vi "Serialize File Attributes.vi"(1 "file attributes":T1 {"permissions" format="%04o"}) -> (0 "Array":u8[](array[numeric]) format="%02x")   [LabVIEW 2020, in "NI_SFTP.lvlib"]
uses:
  <vilib>/net/SFTP/NI_SFTP.lvlib
  <vilib>/net/SFTP/API/Support/File Attributes.ctl
  <vilib>/net/SFTP/Low Level Connection/Serialize U32.vi
  <vilib>/net/SFTP/Low Level Connection/Serialize Byte Array.vi
  <vilib>/net/SFTP/Low Level Connection/Serialize U64.vi
  <vilib>/net/SFTP/Low Level Connection/Low Level Connection.lvclass
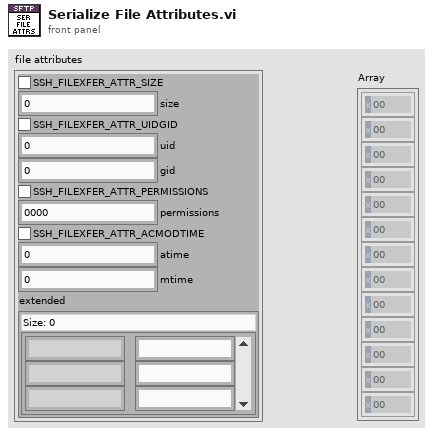
[diagram p1: front panel]
types:
  T1 = typedef "NI_SFTP.lvlib/File Attributes.ctl" = cluster{"SSH_FILEXFER_ATTR_SIZE":bool, "size":u64, "SSH_FILEXFER_ATTR_UIDGID":bool, "uid":u32, "gid":u32, "SSH_FILEXFER_ATTR_PERMISSIONS":bool, "permissions":u32, "SSH_FILEXFER_ATTR_ACMODTIME":bool, "atime":u32, "mtime":u32, "extended":map{string, string}}
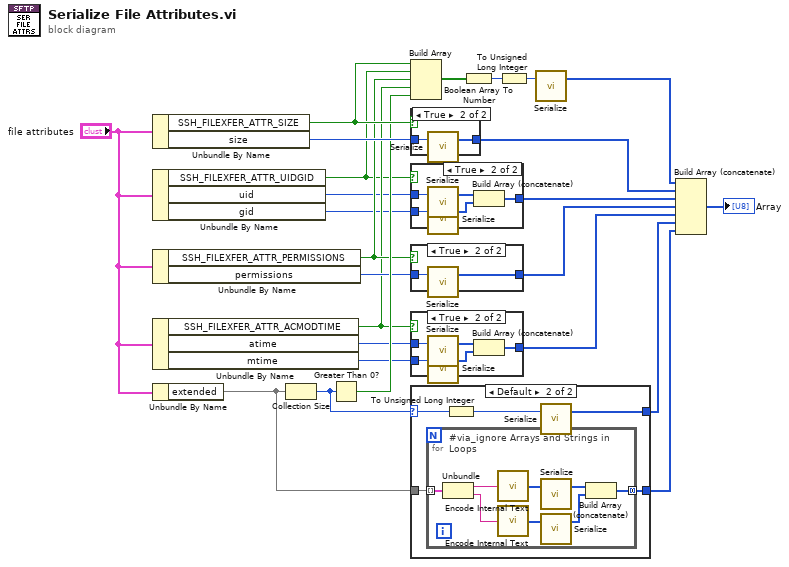
[diagram p0: block diagram]
diagram:
  n1 = Unbundle By Name("file attributes") -> ("SSH_FILEXFER_ATTR_SIZE"=w22:bool, "size"=w21:u64)
  n2 = Unbundle By Name("file attributes") -> ("SSH_FILEXFER_ATTR_UIDGID"=w6:bool, "uid"=w5:u32, "gid"=w4:u32)
  n3 = Unbundle By Name("file attributes") -> ("SSH_FILEXFER_ATTR_PERMISSIONS"=w11:bool, "permissions"=w10:u32)
  n4 = Unbundle By Name("file attributes") -> ("SSH_FILEXFER_ATTR_ACMODTIME"=w9:bool, "atime"=w8:u32, "mtime"=w7:u32)
  n5 = Unbundle By Name("file attributes") -> ("extended"=w12:map{string, string})
  n6 = Collection Size(1:w12) -> (0:w19:i32)
  n7 = Greater Than 0?(x=w19) -> (x > 0?=w20:bool)
  n8 = Build Array(w22, w6, w11, w9, w20) -> (w25:bool[])
  n9 = case shown="True" w22 {
    tunnel: w21 -> [_ w27]
    tunnel: [_ w26] -> w17
    frame False {
    }
    frame True {
      n10 = call-poly <vilib>:"Serialize.vi"("data"=w27) -> ("bytes"=w26:u8[])  [unwired: 2 in]
    }
  }
  n11 = case shown="True" w6 {
    tunnel: w5 -> [_ w32]
    tunnel: [_ w30] -> w16
    tunnel: w4 -> [_ w29]
    frame False {
    }
    frame True {
      n12 = call-poly <vilib>:"Serialize.vi"("data"=w32) -> ("bytes"=w31:u8[])  [unwired: 2 in]
      n13 = call-poly <vilib>:"Serialize.vi"("data"=w29) -> ("bytes"=w28:u8[])  [unwired: 2 in]
      n14 = Build Array (concatenate)(w31, w28) -> (w30:u8[])
    }
  }
  n15 = case shown="True" w11 {
    tunnel: w10 -> [_ w34]
    tunnel: [_ w33] -> w15
    frame False {
    }
    frame True {
      n16 = call-poly <vilib>:"Serialize.vi"("data"=w34) -> ("bytes"=w33:u8[])  [unwired: 2 in]
    }
  }
  n17 = case shown="True" w9 {
    tunnel: w8 -> [_ w39]
    tunnel: [_ w37] -> w14
    tunnel: w7 -> [_ w36]
    frame False {
    }
    frame True {
      n18 = call-poly <vilib>:"Serialize.vi"("data"=w39) -> ("bytes"=w38:u8[])  [unwired: 2 in]
      n19 = call-poly <vilib>:"Serialize.vi"("data"=w36) -> ("bytes"=w35:u8[])  [unwired: 2 in]
      n20 = Build Array (concatenate)(w38, w35) -> (w37:u8[])
    }
  }
  n21 = case shown="Default" w19 {
    selector: w19 -> [_ w41]
    tunnel: w12 -> [_ w44]
    tunnel: [_ w43] -> w2
    tunnel: [_ w42] -> w1
    frame 0 {
    }
    frame Default {
      n22 = for {
        tunnel: w44 -> [w52] mode=indexing
        tunnel: [w49] -> w42 mode=concatenating
        # "#via_ignore Arrays and Strings in Loops"
        n23 = Unbundle(w52) -> (w48:string, w46:string)
        n24 = call <vilib>:"Encode Internal Text.vi"("string"=w48) -> ("data"=w47:u8[])
        n25 = call <vilib>:"Encode Internal Text.vi"("string"=w46) -> ("data"=w45:u8[])
        n26 = call-poly <vilib>:"Serialize.vi"("data"=w47) -> ("bytes"=w51:u8[])  [unwired: 2 in]
        n27 = call-poly <vilib>:"Serialize.vi"("data"=w45) -> ("bytes"=w50:u8[])  [unwired: 2 in]
        n28 = Build Array (concatenate)(w51, w50) -> (w49:u8[])
      }
      n29 = To Unsigned Long Integer(number=w41) -> (unsigned 32bit integer=w40:u32)
      n30 = call-poly <vilib>:"Serialize.vi"("data"=w40) -> ("bytes"=w43:u8[])  [unwired: 2 in]
    }
  }
  n31 = Boolean Array To Number(Boolean array=w25) -> (number=w24:u8)
  n32 = To Unsigned Long Integer(number=w24) -> (unsigned 32bit integer=w23:u32)
  n33 = call-poly <vilib>:"Serialize.vi"("data"=w23) -> ("bytes"=w18:u8[])  [unwired: 2 in]
  n34 = Build Array (concatenate)(w18, w17, w16, w15, w14, w2, w1) -> (→"Array":u8[])
